vi "Flatten EPR and B-Field Arrays.vi"(2 "2D EPR Data":dbl[][](array[numeric]), 3 "2D B-Fields":dbl[][](array[numeric])) -> (0 "1D Flattened EPR Data":dbl[](array[numeric]), 1 "1D Flattened B-Fields":dbl[](array[numeric]))   [LabVIEW 2016]
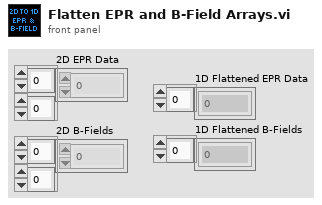
[diagram p1: front panel]
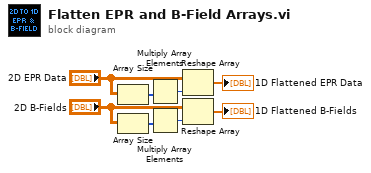
[diagram p0: block diagram]
diagram:
  n1 = Array Size(array="2D EPR Data") -> (size(s)=w8:i32[])
  n2 = Array Size(array="2D B-Fields") -> (size(s)=w4:i32[])
  n3 = Multiply Array Elements(1:w8) -> (0:w7:i32)
  n4 = Multiply Array Elements(1:w4) -> (0:w5:i32)
  n5 = Reshape Array("2D EPR Data", w7) -> (→"1D Flattened EPR Data":dbl[])
  n6 = Reshape Array("2D B-Fields", w5) -> (→"1D Flattened B-Fields":dbl[])
